vi "ledandanalogread.vi"(8 "error in (no error)":errorcluster, 9 "Stop":bool, 10 "Analog Pin":T3, 11 "Arduino Resource in":T1) -> (0 "error out":errorcluster, 1 "Boolean":bool, 2 "Arduino Resource out":T1, 3 "Voltage":dbl(knob) scale=0.0..5.0)   [LabVIEW 2013]
uses:
  <vilib>/LabVIEW Interface for Arduino/Type Defs/Analog Pin.ctl
  <vilib>/LabVIEW Interface for Arduino/Type Defs/Arduino Resource.ctl
  <vilib>/LabVIEW Interface for Arduino/Type Defs/Board Type.ctl
  <vilib>/LabVIEW Interface for Arduino/LabVIEW Interface for Arduino.lvlib
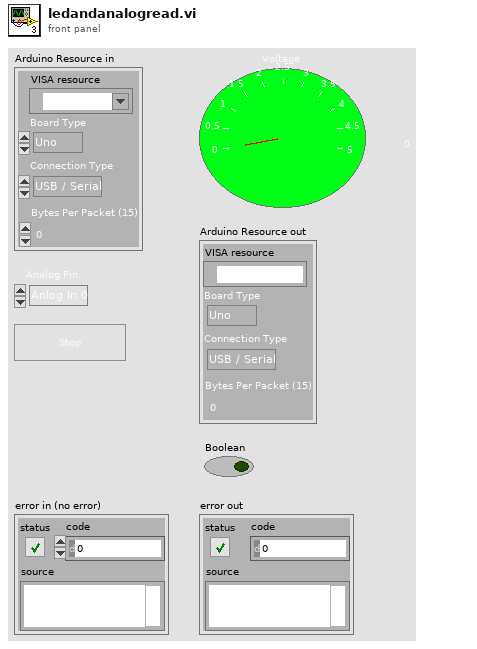
[diagram p1: front panel]
types:
  T1 = typedef "LabVIEW Interface for Arduino.lvlib/Arduino Resource.ctl" = cluster{"VISA resource":refnum<visa-resource-name>, "Board Type":T2, "Connection Type":enum8{"USB / Serial"}, "Bytes Per Packet (15)":u8}
  T2 = typedef "LabVIEW Interface for Arduino.lvlib/Board Type.ctl" = enum16{"Uno", "Dimuelanove w/Atmega 328", "Mega 2560"}
  T3 = typedef "LabVIEW Interface for Arduino.lvlib/Analog Pin.ctl" = enum8{"Anlog In 0", "Anlog In 1", "Anlog In 2", "Anlog In 3", "Anlog In 4", "Anlog In 5"}
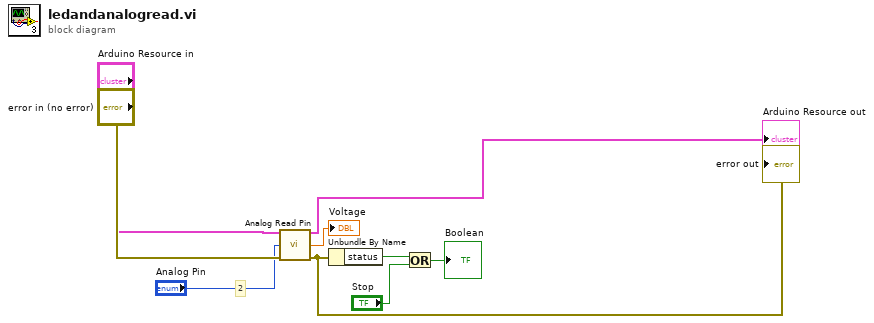
[diagram p0: block diagram]
diagram:
  # "2"
  n1 = call <vilib>:"Analog Read Pin.vi"("Arduino Resource"="Arduino Resource in", "Analog Input Pin (0)"="Analog Pin", "error in"="error in (no error)") -> ("Arduino Resource"=→"Arduino Resource out":T1, "Voltage"=→"Voltage":dbl, "error out"=w8:errorcluster)  [unwired: 10 in]
  "error out" <- w8
  n2 = Unbundle By Name(w8) -> ("status"=w2:bool)
  n3 = Or(x=w2, y="Stop") -> (x .or. y?=→"Boolean":bool)
